vi "Renishaw-XL80_SetResetCompensationMethod.vi"(8 "error in (no error)":errorcluster, 11 "Renishaw-XL80_EMU in":refnum<class "Renishaw-XL80_EMU.lvclass">) -> (0 "error out":errorcluster, 3 "Renishaw-XL80_EMU out":refnum<class "Renishaw-XL80_EMU.lvclass">)   [LabVIEW 2024, in "Renishaw-XL80_EMU.lvclass"]
doc: "This method switches auto-compensation off, returns lambda to its NTP value, and the material compensation factor to 1.\n\nDefinition\nHRESULTResetCompensation();\nParameters\nNone\n\nComments\nThis method always succeeds and returns an HRESULT of S_OK.\n\nIf the client wishes to be compatible with the behaviour of Laser10, then whenever the MeasurementMode is changed to MEASUREMENT_ANGULAR, MEASUREMENT_STRAIGHTNESS_SHORT, or MEASUREMENT_STRAIGHTNESS_LONG then this method should be called in order to turn compensation off."
uses:
  Renishaw-XL80_EMU.lvclass
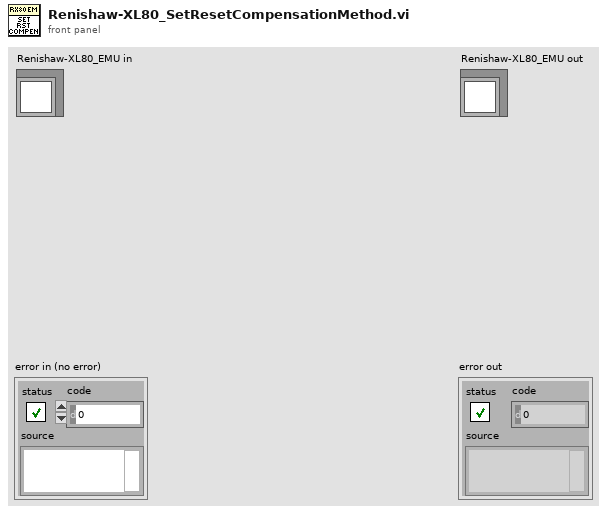
[diagram p1: front panel]
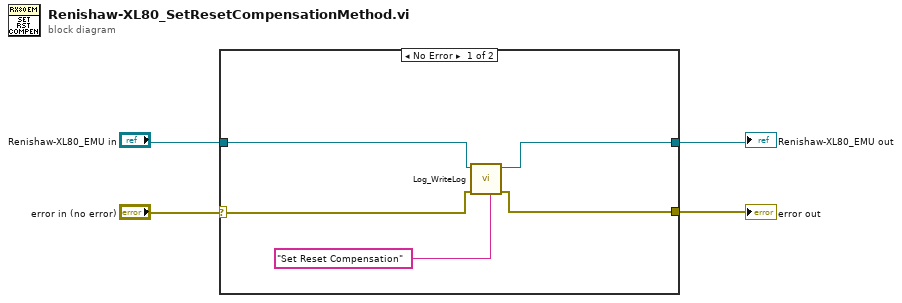
[diagram p0: block diagram]
diagram:
  n1 = case shown="No Error" "error in (no error)" {
    selector: "error in (no error)" -> [w6 w10]
    tunnel: [w8 w11] -> w4
    tunnel: "Renishaw-XL80_EMU in" -> [w9 w11]
    tunnel: [w7 w10] -> w2
    frame No Error {
      n2 = call-dynamic "Log_WriteLog.vi"("Additional text"="Set Reset Compensation", "error in (no error)"=w6, "Log in"=w9) -> ("error out"=w7:errorcluster, "Log out"=w8:refnum<class "Renishaw-XL80_EMU.lvclass">)  [unwired: 7 in]
    }
    frame Error {
    }
  }
  "error out" <- w2
  "Renishaw-XL80_EMU out" <- w4
